vi "Scanner Utility.vi"(8 "error in (no error)":errorcluster, 10 "Message Data":variant, 11 "Data Cluster":T1={"Link"={"Connection"=enum."USB", "Host or IP address (TCP/IP)"="", "Port (Serial/USB)"="COM1"}, "VISA resource"="", "Writer Queue"=refnum, "Status"=FALSE}) -> (0 "error out":errorcluster, 3 "Data Cluster out":T1={"Link"={"Connection"=enum."USB", "Host or IP address (TCP/IP)"="", "Port (Serial/USB)"="COM1"}, "VISA resource"="", "Writer Queue"=refnum, "Status"=FALSE})   [LabVIEW 2020, in "Hiden Scanner.lvlib"]
uses:
  Hiden Scanner.lvlib
  Scanner Hardware Configuration.ctl
  support/Message Queue/Message Cluster.ctl
  support/Message Queue/Message Queue.lvlib
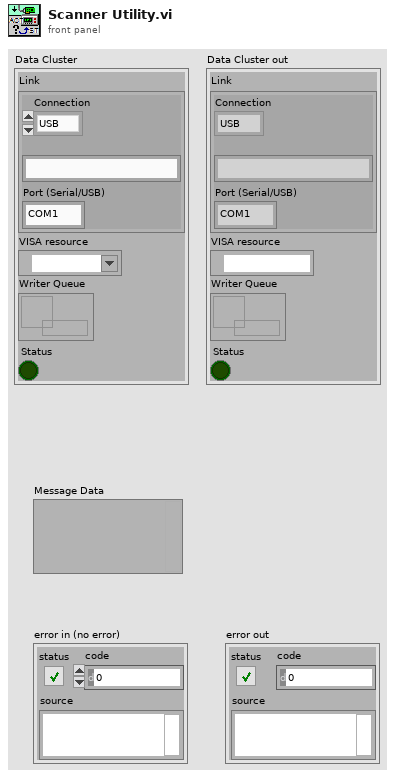
[diagram p1: front panel]
types:
  T1 = typedef "Hiden Scanner.lvlib/Scanner Hardware Configuration.ctl" = cluster{"Link":cluster{"Connection":enum16{"Serial", "TCP/IP", "USB"}, "Host or IP address (TCP/IP)":string, "Port (Serial/USB)":string}, "VISA resource":refnum<visa-resource-name>, "Writer Queue":refnum<queue>, "Status":bool}
  T2 = typedef "Message Queue.lvlib/Message Cluster.ctl" = cluster{"Message":string, "Message Data":variant}
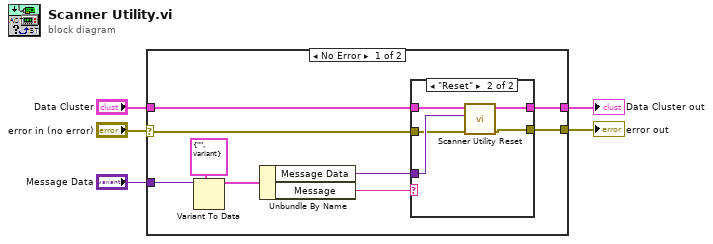
[diagram p0: block diagram]
diagram:
  n1 = case shown="No Error" "error in (no error)" {
    selector: "error in (no error)" -> [w7 w22]
    tunnel: [w14 w22] -> w5
    tunnel: "Data Cluster" -> [w13 w23]
    tunnel: [w12 w23] -> w3
    tunnel: "Message Data" -> [w8 _]
    frame No Error {
      n2 = Variant To Data(type=T2 {"Message"="", "Message Data"=variant} ("element"), Variant=w8) -> (data=w10:T2)  [unwired: 1 in, 1 out]
      n3 = Unbundle By Name(w10) -> ("Message Data"=w6:variant, "Message"=w11:string)
      n4 = case shown="\"Reset\"" w11 {
        tunnel: w6 -> [_ w20]
        tunnel: [w16 w17] -> w12
        tunnel: w13 -> [w16 w21]
        tunnel: w7 -> [w15 w19]
        tunnel: [w15 w18] -> w14
        frame "False", Default {
        }
        frame "Reset" {
          n5 = call "Scanner Utility Reset.vi"("error in (no error)"=w19, "Message Data"=w20, "Data Cluster in"=w21) -> ("error out"=w18:errorcluster, "Data Cluster out"=w17:T1)  [unwired: 7 in]
        }
      }
    }
    frame Error {
    }
  }
  "error out" <- w5
  "Data Cluster out" <- w3
